vi "Read_TDMS_Data.vi"(5 "offset (0)":i64, 7 "count (-1: all)":i64, 10 "Listbox":i32[](array[numeric])) -> (0 "Properties":dbl[][](array[numeric]), 3 "Data":T1(array[cluster]))   [LabVIEW 2017]
uses:
  <vilib>/Utility/error.llb/DialogType.ctl
  Data_Analysis_Global_var.vi
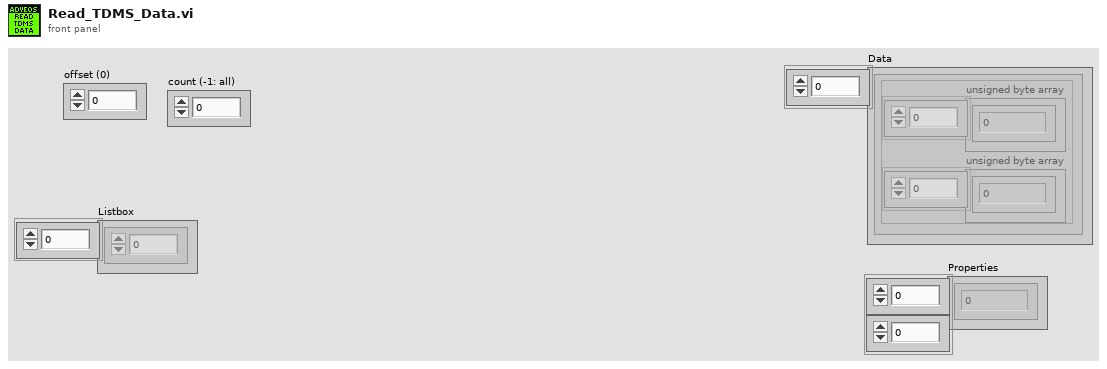
[diagram p1: front panel]
types:
  T1 = cluster{"unsigned byte array":i32[], "unsigned byte array":i32[]}[]
  T2 = typedef "DialogType.ctl" = u16
  T3 = cluster{"unsigned byte array":i32[], "unsigned byte array":i32[]}
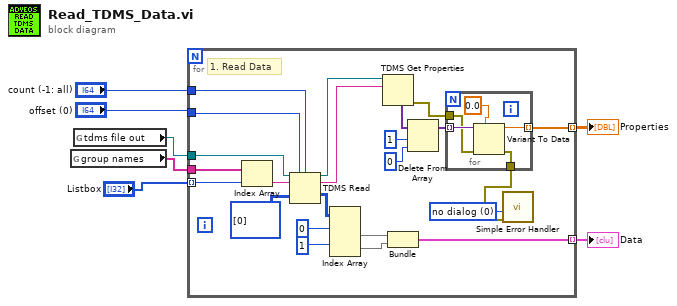
[diagram p0: block diagram]
diagram:
  n1 = global read "Data_Analysis_Global_var.vi" "group names"() -> (w3:string[])
  n2 = global read "Data_Analysis_Global_var.vi" "tdms file out"() -> (w4:refnum<k34>)
  n3 = for {
    tunnel: "Listbox" -> [w30] mode=indexing
    tunnel: "count (-1: all)" -> [w25]
    tunnel: "offset (0)" -> [w24]
    tunnel: w4 -> [w23]
    tunnel: w3 -> [w22]
    tunnel: [w20] -> w2 mode=indexing
    tunnel: [w8] -> w1 mode=indexing
    w13 = T2 0 items=["no dialog", "OK message", "continue or stop message", "OK message + warnings", "continue/stop + warnings"] ("type of dialog (OK msg:1)")
    # "1. Read Data"
    n4 = Index Array(array=w22, index=w30) -> (element=w21:string)
    n5 = TDMS Read(0:w23, 1:w24, 2:w25, 5:w21, 12:i32[][] [[0]] ("unsigned byte array")) -> (4:w10:refnum<k34>, 6:w9:string, 10:w26:i32[][])  [unwired: 3 in, 3 out]
    n6 = Index Array(array=w26, index (row) #1=0 ("index (row)"), index (row) #2=1 ("index (row)")) -> (element #1=w19:i32[], element #2=w18:i32[])  [unwired: 2 in]
    n7 = TDMS Get Properties(10:w9, 11:w10) -> (0:w16:errorcluster, 4:w15:variant[])  [unwired: 2 in, 6 out]
    n8 = Bundle("unsigned byte array"=w19, "unsigned byte array"=w18) -> (w20:T3)  [unwired: 1 in]
    n9 = Delete From Array(array=w15, length=1, index=0 ("length")) -> (array with subset deleted=w14:variant[])  [unwired: 1 out]
    n10 = for {
      tunnel: [w35] -> w8 mode=indexing
      tunnel: w14 -> [w34] mode=indexing
      tunnel: [w32] -> w17
      tunnel: w16 -> [w31]
      n11 = Variant To Data(error in=w31, type=0.0, Variant=w34) -> (data=w35:dbl, error out=w32:errorcluster)
    }
    n12 = call <vilib>:"Simple Error Handler.vi"("type of dialog (OK msg:1)"=w13, "error in (no error)"=w17) -> ()  [unwired: 3 in, 5 out]
  }
  "Data" <- w2
  "Properties" <- w1
